vi "subvi_load_data_vector.vi"(11 "default name":path) -> (3 "array type (2D Dbl) out":dbl[](array[numeric]))   [LabVIEW 2020]
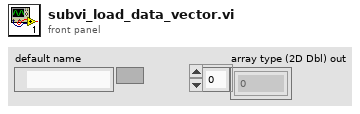
[diagram p1: front panel]
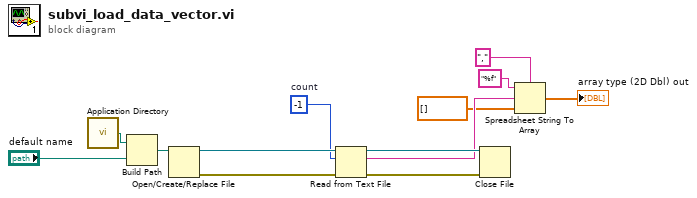
[diagram p0: block diagram]
diagram:
  w2 = -1  # count
  n1 = call <vilib>:"Application Directory.vi"() -> ("Application Directory"=w6:path)
  n2 = Build Path(base path=w6, name or relative path="default name") -> (appended path=w5:path)
  n3 = Open/Create/Replace File(file path (use dialog)=w5) -> (refnum out=w10:refnum<file>, error out=w11:errorcluster)  [unwired: 5 in, 1 out]
  n4 = Read from Text File(file (use dialog)=w10, count=w2, error in=w11) -> (refnum out=w9:refnum<file>, text=w7:string, error out=w8:errorcluster)  [unwired: 1 in, 1 out]
  n5 = Close File(refnum=w9, error in=w8) -> ()  [unwired: 2 out]
  n6 = Spreadsheet String To Array(delimiter (Tab)=",", format string="%f", spreadsheet string=w7, array type (2D Dbl)=dbl[] []) -> (array=→"array type (2D Dbl) out":dbl[])
